vi "S2C_XML_Close.vi"(8 "Error In":errorcluster) -> (0 "Error Out":errorcluster)   [LabVIEW 2015]
uses:
  S2C_XML_Globals.vi
  <vilib>/xml/Close Reference(Node).vi
  <vilib>/xml/NI_XML.lvlib
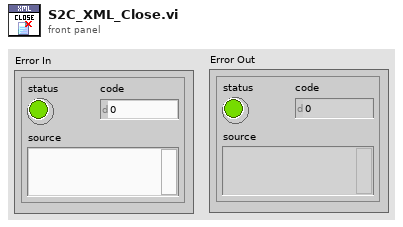
[diagram p1: front panel]
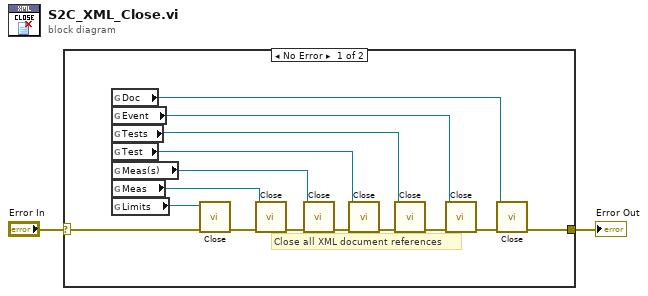
[diagram p0: block diagram]
diagram:
  n1 = case shown="No Error" "Error In" {
    selector: "Error In" -> [w8 w18]
    tunnel: [w3 w18] -> w1
    frame No Error {
      # "Close all XML document references"
      n2 = global read "S2C_XML_Globals.vi" "Doc"() -> (w4:refnum<k20>)
      n3 = global read "S2C_XML_Globals.vi" "Event"() -> (w17:refnum<k20>)
      n4 = global read "S2C_XML_Globals.vi" "Tests"() -> (w16:refnum<k20>)
      n5 = global read "S2C_XML_Globals.vi" "Test"() -> (w14:refnum<k20>)
      n6 = global read "S2C_XML_Globals.vi" "Meas(s)"() -> (w10:refnum<k20>)
      n7 = global read "S2C_XML_Globals.vi" "Meas"() -> (w9:refnum<k20>)
      n8 = global read "S2C_XML_Globals.vi" "Limits"() -> (w6:refnum<k20>)
      n9 = call-poly <vilib>:"Close.vi"("error in (no error)"=w8, "node"=w6) -> ("error out"=w7:errorcluster)  [unwired: 7 in]
      n10 = call-poly <vilib>:"Close.vi"("error in (no error)"=w7, "node"=w9) -> ("error out"=w12:errorcluster)  [unwired: 7 in]
      n11 = call-poly <vilib>:"Close.vi"("error in (no error)"=w12, "node"=w10) -> ("error out"=w11:errorcluster)  [unwired: 7 in]
      n12 = call-poly <vilib>:"Close.vi"("error in (no error)"=w11, "node"=w14) -> ("error out"=w13:errorcluster)  [unwired: 7 in]
      n13 = call-poly <vilib>:"Close.vi"("error in (no error)"=w13, "node"=w16) -> ("error out"=w15:errorcluster)  [unwired: 7 in]
      n14 = call-poly <vilib>:"Close.vi"("error in (no error)"=w15, "node"=w17) -> ("error out"=w5:errorcluster)  [unwired: 7 in]
      n15 = call-poly <vilib>:"Close.vi"("error in (no error)"=w5, "node"=w4) -> ("error out"=w3:errorcluster)  [unwired: 7 in]
    }
    frame Error {
    }
  }
  "Error Out" <- w1
